vi "WaitMsecs pause if key hit.vi"(8 "error in (no error)":errorcluster, 11 "Wait Msecs":dbl) -> (0 "error out":errorcluster)   [LabVIEW 2013]
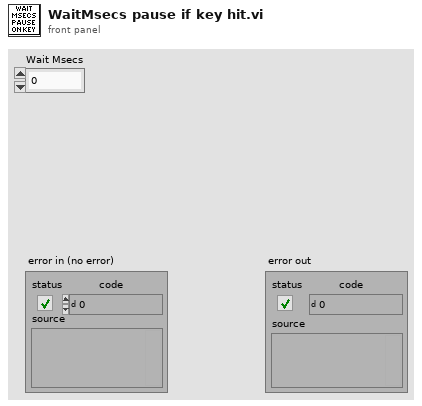
[diagram p1: front panel]
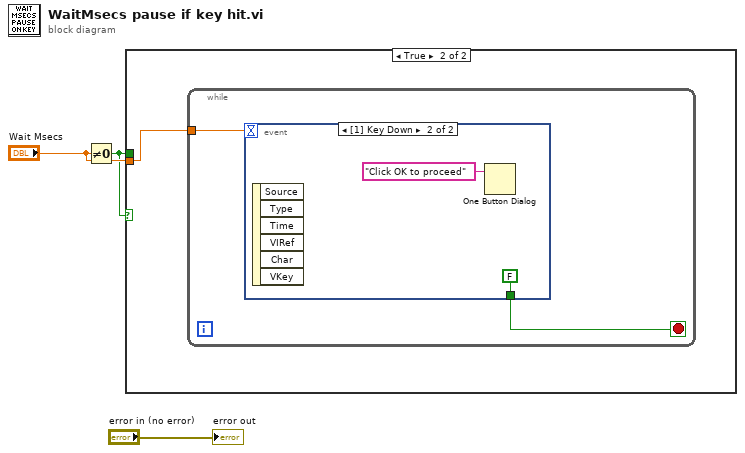
[diagram p0: block diagram]
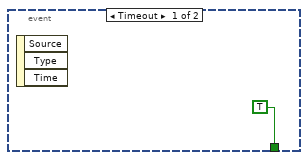
[diagram p3: hidden frame]
diagram:
  n1 = Not Equal To 0?(x="Wait Msecs") -> (x != 0?=w1:bool)
  n2 = case shown="True" w1 {
    tunnel: "Wait Msecs" -> [_ w4]
    tunnel: w1 -> [_ _]
    frame False {
    }
    frame True {
      n3 = while {
        tunnel: w4 -> [w6]
        stop <- w5 stop-if-true
        n4 = event shown="[1] Key Down" {
          selector: _ -> [_ _]
          dyn-events: _ -> [_ _]
          timeout: w6 -> [_ _]
          tunnel: [TRUE FALSE] -> w5
          event Timeout {
            n5 = event-data() -> ()  [unwired: 1 in, 3 out]
          }
          event Key Down {
            n6 = event-data() -> ()  [unwired: 1 in, 6 out]
            n7 = One Button Dialog(message="Click OK to proceed") -> ()  [unwired: 1 in, 1 out]
          }
        }
      }
    }
  }
  "error out" <- "error in (no error)"
